vi "IntuitiveSteering_theta.vi"(0 "Input":dbl, 5 "Forward Time":dbl, 7 "Phase Shift":dbl, 9 "Max. Amplitude":dbl) -> (4 "Servo Position":T1)   [LabVIEW 2013]
uses:
  My Computer/Controls/Servo Position.ctl
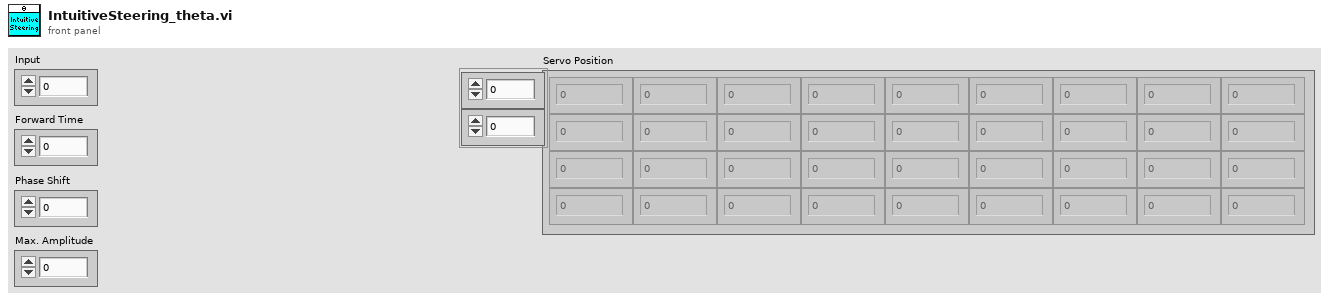
[diagram p1: front panel]
types:
  T1 = typedef "Servo Position.ctl" = dbl[][]
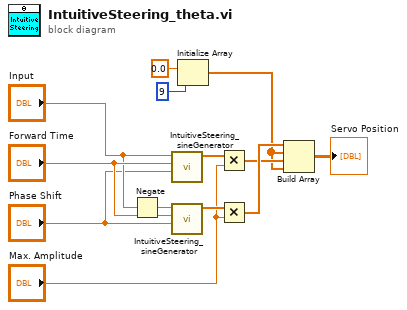
[diagram p0: block diagram]
diagram:
  n1 = Negate(x="Input") -> (-x=w13:dbl)
  n2 = call "IntuitiveSteering_sineGenerator.vi"("Phase Shift"="Phase Shift", "Forward Time"="Forward Time", "Input"="Input") -> ("Fin Position"=w8:dbl[])  [unwired: 8 in]
  n3 = call "IntuitiveSteering_sineGenerator.vi"("Phase Shift"="Phase Shift", "Forward Time"="Forward Time", "Input"=w13) -> ("Fin Position"=w9:dbl[])  [unwired: 8 in]
  n4 = Initialize Array(0.0 ("element"), 9 ("dimension size")) -> (w2:dbl[])
  n5 = Multiply(x=w8, y="Max. Amplitude") -> (x*y=w5:dbl[])
  n6 = Multiply(x=w9, y="Max. Amplitude") -> (x*y=w6:dbl[])
  n7 = Build Array(w6, w2, w5, w2) -> (→"Servo Position":dbl[][])
